vi "CAN Start Engine.vi"(9 "ECU CAN Port":string, 11 "Sequence Context":T1) -> (0 "error out":errorcluster)   [LabVIEW 2023, in "LTT_TeststandSteptypes.lvlib"]
uses:
  LTT_TeststandSteptypes.lvlib
  <vilib>/addons/TestStand/_TSLegacy.llb/LabVIEW Test - Sequence Context.ctl
  Control/CAN FGV State.ctl
  HardwareAbstractionLayer_LVOOP/CAN/CAN Lib/NI-XNET_class/NI-XNET.lvclass
  HardwareAbstractionLayer_LVOOP/Teststand/Teststand.lvclass
  HardwareAbstractionLayer_LVOOP/CAN/CAN Application Protocols/STP Protocol_class/STP Protocol.lvclass
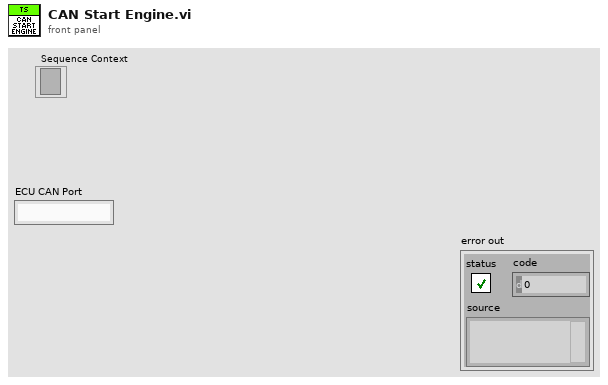
[diagram p1: front panel]
types:
  T1 = typedef "LabVIEW Test - Sequence Context.ctl" = refnum<k7>
  T2 = typedef "HardwareAbstractionLayer_LVOOP.lvlib/Teststand.lvclass/Teststand Status Control.ctl" = cluster{"Terminating or Aborting":bool, "Stop":bool, "Socket Count":i16, "Selected Sockets":i16[]}
  T3 = typedef "LTT_TeststandSteptypes.lvlib/CAN FGV State.ctl" = enum16{"Init", "Get", "Set"}
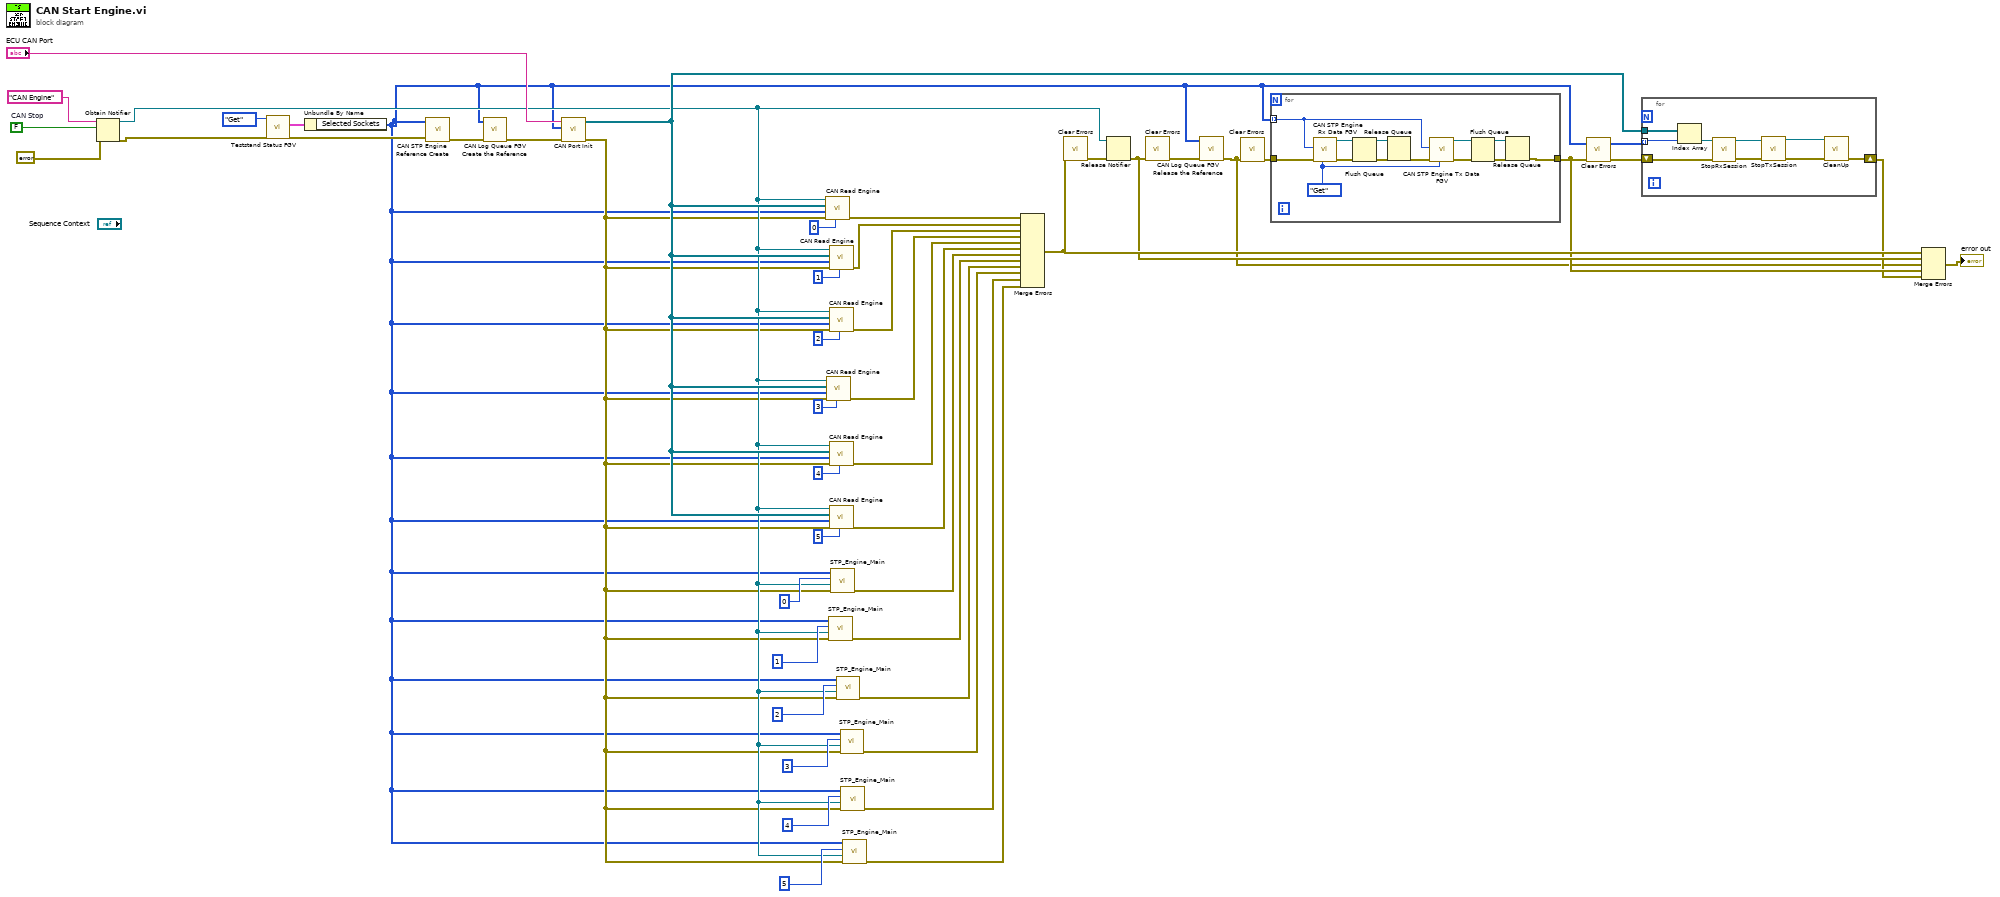
[diagram p0: block diagram]
diagram:
  w44 = FALSE  # CAN Stop
  n1 = Obtain Notifier(name (unnamed)="CAN Engine", notification data type=w44, error in (no error)=errorcluster {"status"=FALSE, "code"=0, "source"=""}) -> (notifier out=w21:refnum<notifier>, error out=w13:errorcluster)  [unwired: 1 in, 1 out]
  n2 = call "Teststand Status FGV.vi"("error in"=w13, "Option"=enum16{"Set", "Get"}."Get") -> ("error out"=w12:errorcluster, "Teststand Status Out"=w48:T2)  [unwired: 8 in]
  n3 = Unbundle By Name(w48) -> ("Selected Sockets"=w3:i16[])
  n4 = call "CAN STP Engine Reference Create.vi"("error in"=w12, "Selected Sockets"=w3) -> ("error out"=w6:errorcluster)  [unwired: 9 in]
  n5 = call "CAN Log Queue FGV Create the Reference.vi"("error in"=w6, "Selected Sockets"=w3) -> ("error out"=w5:errorcluster)  [unwired: 9 in]
  n6 = call "CAN Port Init.vi"("error in (no error)"=w5, "Selected Sockets"=w3, "ECU CAN Port"="ECU CAN Port") -> ("error out"=w20:errorcluster, "CAN Ref Out"=w31:refnum<class "NI-XNET.lvclass">[])  [unwired: 7 in]
  n7 = call "CAN Read Engine.vi"("Current Scoket"=i16 0, "error in (no error)"=w20, "Selected Sockets"=w3, "CAN Ref Out"=w31, "Notifier in"=w21) -> ("error out"=w43:errorcluster)  [unwired: 6 in]
  n8 = call "CAN Read Engine.vi"("Current Scoket"=i16 3, "error in (no error)"=w20, "Selected Sockets"=w3, "CAN Ref Out"=w31, "Notifier in"=w21) -> ("error out"=w34:errorcluster)  [unwired: 6 in]
  n9 = call "STP_Engine_Main.vi"("error in"=w20, "notifier in"=w21, "Socket No"=i16 1 ("Current Scoket"), "Selected Sockets"=w3) -> ("error out"=w18:errorcluster)  [unwired: 7 in]
  n10 = call "CAN Read Engine.vi"("Current Scoket"=i16 1, "error in (no error)"=w20, "Selected Sockets"=w3, "CAN Ref Out"=w31, "Notifier in"=w21) -> ("error out"=w36:errorcluster)  [unwired: 6 in]
  n11 = call "CAN Read Engine.vi"("Current Scoket"=i16 2, "error in (no error)"=w20, "Selected Sockets"=w3, "CAN Ref Out"=w31, "Notifier in"=w21) -> ("error out"=w35:errorcluster)  [unwired: 6 in]
  n12 = call "CAN Read Engine.vi"("Current Scoket"=i16 4, "error in (no error)"=w20, "Selected Sockets"=w3, "CAN Ref Out"=w31, "Notifier in"=w21) -> ("error out"=w33:errorcluster)  [unwired: 6 in]
  n13 = call "CAN Read Engine.vi"("Current Scoket"=i16 5, "error in (no error)"=w20, "Selected Sockets"=w3, "CAN Ref Out"=w31, "Notifier in"=w21) -> ("error out"=w32:errorcluster)  [unwired: 6 in]
  n14 = call "STP_Engine_Main.vi"("error in"=w20, "notifier in"=w21, "Socket No"=i16 0 ("Current Scoket"), "Selected Sockets"=w3) -> ("error out"=w19:errorcluster)  [unwired: 7 in]
  n15 = call "STP_Engine_Main.vi"("error in"=w20, "notifier in"=w21, "Socket No"=i16 2 ("Current Scoket"), "Selected Sockets"=w3) -> ("error out"=w17:errorcluster)  [unwired: 7 in]
  n16 = call "STP_Engine_Main.vi"("error in"=w20, "notifier in"=w21, "Socket No"=i16 3 ("Current Scoket"), "Selected Sockets"=w3) -> ("error out"=w16:errorcluster)  [unwired: 7 in]
  n17 = call "STP_Engine_Main.vi"("error in"=w20, "notifier in"=w21, "Socket No"=i16 4 ("Current Scoket"), "Selected Sockets"=w3) -> ("error out"=w15:errorcluster)  [unwired: 7 in]
  n18 = call "STP_Engine_Main.vi"("error in"=w20, "notifier in"=w21, "Socket No"=i16 5 ("Current Scoket"), "Selected Sockets"=w3) -> ("error out"=w14:errorcluster)  [unwired: 7 in]
  n19 = Merge Errors(w43, w36, w35, w34, w33, w32, w19, w18, w17, w16, w15, w14) -> (w10:errorcluster)
  n20 = call <vilib>:"Clear Errors.vi"("error in (no error)"=w10) -> ("error out"=w28:errorcluster)  [unwired: 5 in, 1 out]
  n21 = Release Notifier(notifier=w21, error in (no error)=w28) -> (error out=w9:errorcluster)  [unwired: 1 in, 2 out]
  n22 = call <vilib>:"Clear Errors.vi"("error in (no error)"=w9) -> ("error out"=w4:errorcluster)  [unwired: 5 in, 1 out]
  n23 = call "CAN Log Queue FGV Release the Reference.vi"("error in"=w4, "Selected Sockets"=w3) -> ("error out"=w2:errorcluster)  [unwired: 9 in]
  n24 = call <vilib>:"Clear Errors.vi"("error in (no error)"=w2) -> ("error out"=w1:errorcluster)  [unwired: 5 in, 1 out]
  n25 = for {
    tunnel: w1 -> [w61]
    tunnel: w3 -> [w60] mode=indexing
    tunnel: [w51] -> w8
    w59 = CAN_FGV_State."Get" ("CAN FGV State")
    n26 = call "CAN STP Engine Rx Data FGV.vi"("CAN FGV State"=w59, "error in"=w61, "Socket No"=w60) -> ("error out"=w57:errorcluster, "STP Engine Rx Data Out"=w58:refnum<queue>)  [unwired: 7 in]
    n27 = Flush Queue(queue=w58, error in (no error)=w57) -> (queue out=w55:refnum<queue>, error out=w56:errorcluster)  [unwired: 1 out]
    n28 = Release Queue(queue=w55, error in (no error)=w56) -> (error out=w53:errorcluster)  [unwired: 1 in, 2 out]
    n29 = call "CAN STP Engine Tx Data FGV.vi"("CAN FGV State"=w59, "error in"=w53, "Socket No"=w60) -> ("error out"=w52:errorcluster, "STP Engine Tx Data out"=w49:refnum<queue>)  [unwired: 6 in, 1 out]
    n30 = Flush Queue(queue=w49, error in (no error)=w52) -> (queue out=w54:refnum<queue>, error out=w50:errorcluster)  [unwired: 1 out]
    n31 = Release Queue(queue=w54, error in (no error)=w50) -> (error out=w51:errorcluster)  [unwired: 1 in, 2 out]
  }
  n32 = call <vilib>:"Clear Errors.vi"("error in (no error)"=w8) -> ("error out"=w11:errorcluster)  [unwired: 5 in, 1 out]
  n33 = for {
    tunnel: w31 -> [w64]
    tunnel: w3 -> [w63] mode=indexing
    shift-right: [w65] -> w7
    shift-left: w11 -> [w66]
    n34 = Index Array(array=w64, index=w63) -> (element=w62:refnum<class "NI-XNET.lvclass">)
    n35 = call-dynamic "StopRxSession.vi"("error in (no error)"=w66, "NI-XNET in"=w62) -> ("error out"=w69:errorcluster, "NI-XNET out"=w70:refnum<class "NI-XNET.lvclass">)  [unwired: 8 in]
    n36 = call-dynamic "StopTxSession.vi"("error in (no error)"=w69, "NI-XNET in"=w70) -> ("error out"=w68:errorcluster, "NI-XNET out"=w67:refnum<class "NI-XNET.lvclass">)  [unwired: 8 in]
    n37 = call-dynamic "CleanUp.vi"("object in"=w67, "error in (no error)"=w68) -> ("error out"=w65:errorcluster)  [unwired: 12 in, 1 out]
  }
  n38 = Merge Errors(w10, w9, w2, w8, w7) -> (→"error out":errorcluster)
